vi "sub1.vi"(2 "정지 In":bool, 3 "데이터 In":dbl, 4 "FGV 상태":enum16{"쓰기", "읽기"}(ring)) -> (0 "정지 Out":bool, 1 "데이터 Out":dbl)   [LabVIEW 2020]
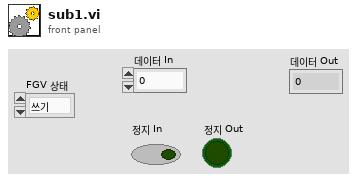
[diagram p1: front panel]
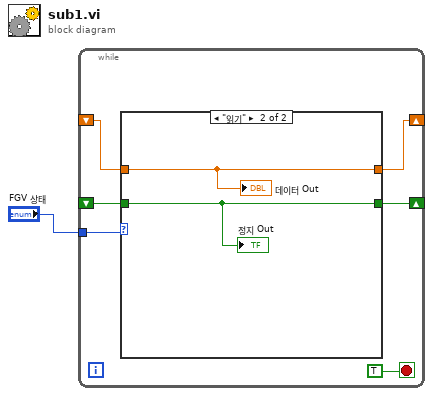
[diagram p0: block diagram]
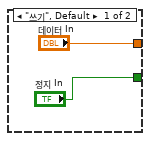
[diagram p2: hidden frame]
diagram:
  n1 = while {
    shift-right: [w6] -> _
    shift-left: _ -> [w4]
    shift-right: [w5] -> _
    shift-left: _ -> [w3]
    tunnel: "FGV 상태" -> [w7]
    stop <- TRUE stop-if-true
    n2 = case shown="\"읽기\"" w7 {
      tunnel: ["데이터 In" w11] -> w6
      tunnel: ["정지 In" w10] -> w5
      tunnel: w4 -> [_ w11]
      tunnel: w3 -> [_ w10]
      frame "쓰기", Default {
      }
      frame "읽기" {
        "정지 Out" <- w10
        "데이터 Out" <- w11
      }
    }
  }
